vi "getShortStatus.vi"(8 "error in (no error)":errorcluster, 11 "DomeCommunicator in":refnum<class "ATDomeCommunicator.lvclass">) -> (0 "error out":errorcluster, 1 "timeout":bool, 2 "shortStatus out":T1 {"azimuthAngle" min=0.0 max=360.0; "dropoutDoorOpeningPercentage" min=0.0 max=100.0; "mainDoorOpeningPercentage" min=0.0 max=100.0}, 3 "DomeCommunicator out":refnum<class "ATDomeCommunicator.lvclass">, 4 "response":string)   [LabVIEW 2016, in "ATDomeCommunicator.lvclass"]
uses:
  ATDomeCommunicator.lvclass
  ComTypedefs/shortStatus.ctl
  ComTypedefs/openingStates.ctl
  IDome/domeTypedefs/openingPercentage.ctl
  ComTypedefs/sensorCode.ctl
  ComTypedefs/azimimuthPositionStatus.ctl
  IDome/domeTypedefs/azimuth.ctl
  IDome/domeTypedefs/direction.ctl
  IDome/domeTypedefs/domeState.ctl
  IDome/domeTypedefs/motionDirection.ctl
  IDome/domeTypedefs/openingMotion.ctl
  ComTypedefs/queries.ctl
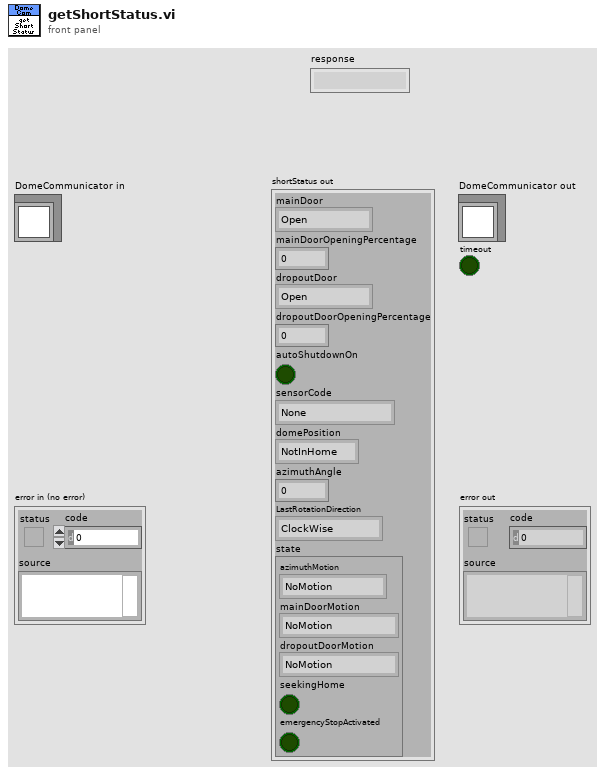
[diagram p1: front panel]
types:
  T1 = typedef "shortStatus.ctl" = cluster{"mainDoor":T2, "mainDoorOpeningPercentage":T3, "dropoutDoor":T2, "dropoutDoorOpeningPercentage":T3, "autoShutdownOn":bool, "sensorCode":T4, "domePosition":T5, "azimuthAngle":T6, "LastRotationDirection":T7, "state":T8}
  T2 = typedef "openingStates.ctl" = enum16{"Open", "Shut", "Ajar"}
  T3 = typedef "openingPercentage.ctl" = dbl
  T4 = typedef "sensorCode.ctl" = enum16{"None", "RainSnowSensorTriggered", "CloudSensorTriggered", "BothSensorsTriggered"}
  T5 = typedef "azimimuthPositionStatus.ctl" = enum16{"NotInHome", "Home"}
  T6 = typedef "azimuth.ctl" = dbl
  T7 = typedef "direction.ctl" = enum16{"ClockWise", "CounterClockWise"}
  T8 = typedef "domeState.ctl" = cluster{"azimuthMotion":T9, "mainDoorMotion":T10, "dropoutDoorMotion ":T10, "seekingHome":bool, "emergencyStopActivated":bool}
  T9 = typedef "motionDirection.ctl" = enum16{"NoMotion", "MovingClockWise", "MovingCounterClockWise"}
  T10 = typedef "openingMotion.ctl" = enum16{"NoMotion", "Opening", "Closing"}
  T11 = typedef "queries.ctl" = enum16{"ShortStatus", "FullEngineeringStatus", "RecallLastSavedConfiguration"}
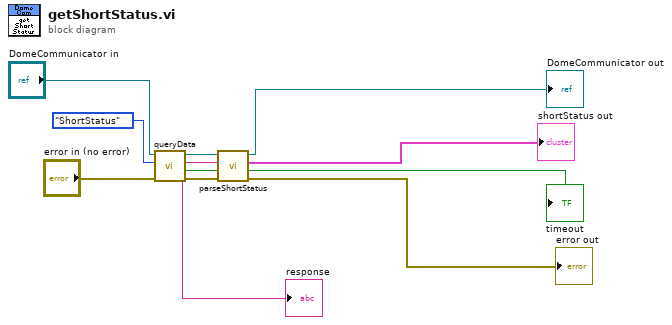
[diagram p0: block diagram]
diagram:
  n1 = call "queryData.vi"("error in (no error)"="error in (no error)", "queries"=queries."ShortStatus", "DomeCommunicator in"="DomeCommunicator in") -> ("error out"=w5:errorcluster, "timeout"=→"timeout":bool, "response"=w4:string, "DomeCommunicator out"=w7:refnum<class "ATDomeCommunicator.lvclass">)  [unwired: 5 in]
  "response" <- w4
  n2 = call "parseShortStatus.vi"("error in (no error)"=w5, "shortStatusString"=w4, "DomeCommunicator in"=w7) -> ("error out"=→"error out":errorcluster, "shortStatus out"=→"shortStatus out":T1, "DomeCommunicator out"=→"DomeCommunicator out":refnum<class "ATDomeCommunicator.lvclass">)  [unwired: 6 in]
